vi "M266 VI Tester.vi"() -> ()   [LabVIEW 2014]
panel:
  out "Dispersion":dbl format="%.4f"
  in  "Demo mode":bool=TRUE
  out "Error":string
  out "Cur. state":i32(ring) items=["Unknown", "Open", "Close"]
  in  "Set shutter state":bool
  in  "Select shutter state":u32(ring) items=["Open", "Close"]
  out "Cur. filter":i32(ring) items=["Filter1", "Filter2", "Filter3", "Filter4", "Filter5", "Filter6", "Filter7", "Filter8"]
  in  "Set filter":bool
  in  "Select filter":i32(ring) items=["Filter1", "Filter2", "Filter3", "Filter4", "Filter5", "Filter6", "Filter7", "Filter8"]
  out "Cur. mirror":u32(ring) items=["Axial port", "Lateral port"]
  in  "Set mirror":bool
  in  "Select mirror":i32(ring) items=["Axial port", "Lateral port"]
  in  "Reset":bool
  in  "Set slit width":bool
  out "Slit width":dbl format="%.2f"
  in  "Select slit":u32(ring) items=["Entrance Slit", "Exit Slit"]
  in  "New slit width":dbl format="%.2f"
  in  "Stop control":bool
  in  "Reset":bool caption="bReset"
  in  "Set new WL":bool caption="Boolean"
  out "Cur WL":dbl format="%.2f"
  in  "New WL":dbl format="%.2f"
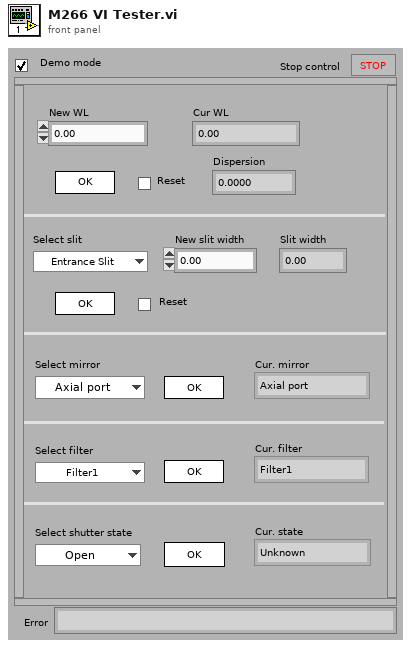
[diagram p1: front panel]
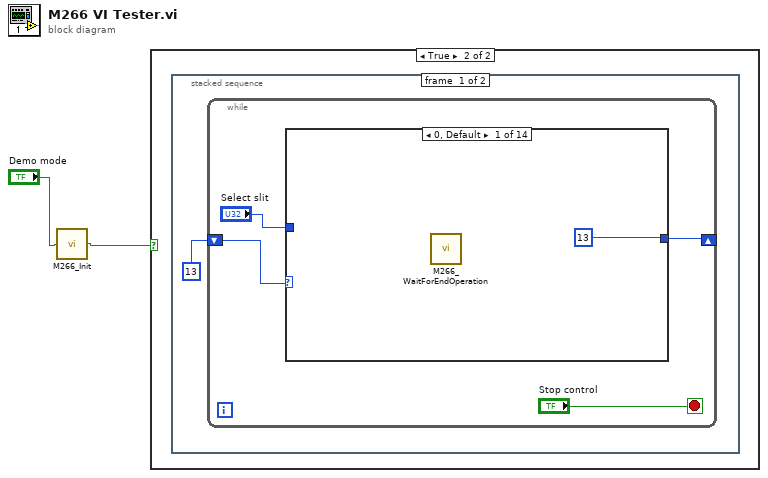
[diagram p0: block diagram]
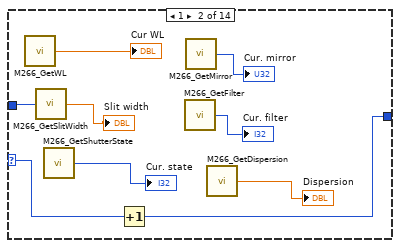
[diagram p3: hidden frame]
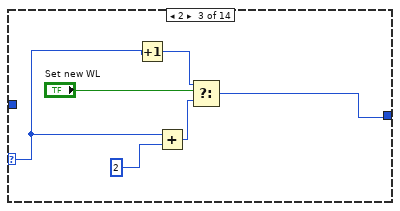
[diagram p4: hidden frame]
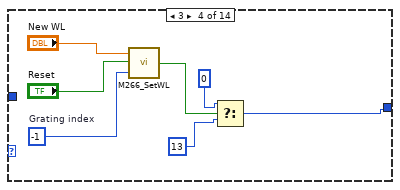
[diagram p5: hidden frame]
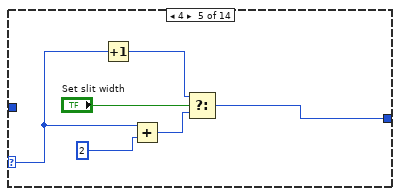
[diagram p6: hidden frame]
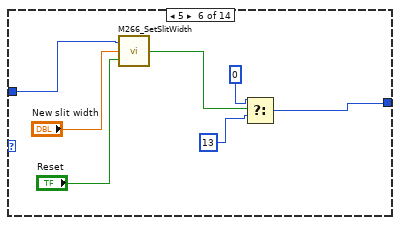
[diagram p7: hidden frame]
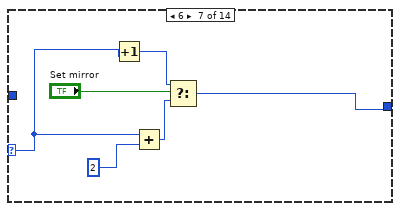
[diagram p8: hidden frame]
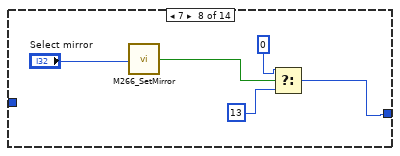
[diagram p9: hidden frame]
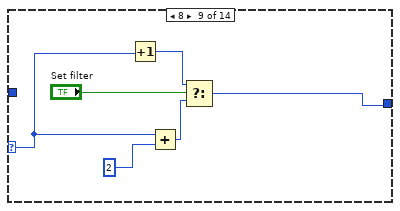
[diagram p10: hidden frame]
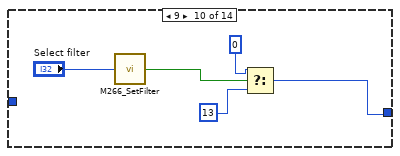
[diagram p11: hidden frame]
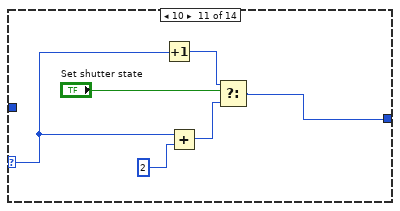
[diagram p12: hidden frame]
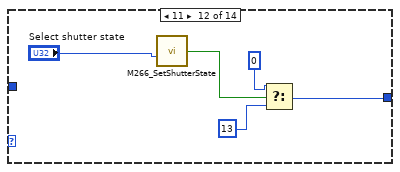
[diagram p13: hidden frame]
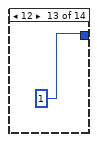
[diagram p14: hidden frame]
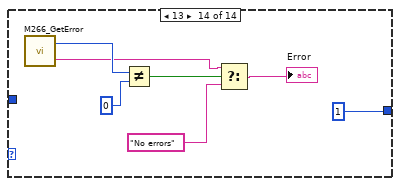
[diagram p15: hidden frame]
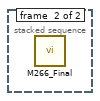
[diagram p16: hidden frame]
diagram:
  n1 = call "M266_Init.vi"("Demo mode"="Demo mode") -> ("Result"=w1:bool)
  n2 = case shown="True" w1 {
    frame False {
    }
    frame True {
      n3 = stacked-sequence {
        frame #0 {
          n4 = while {
            shift-right: [w5] -> _
            shift-left: 13 -> [w4]
            stop <- "Stop control" stop-if-true
            n5 = case shown="0, Default" w4 {
              selector: w4 -> [_ w13 w18 _ w31 _ w45 _ w56 _ w69 _ _ _]
              tunnel: "Select slit" -> [_ w15 _ _ _ w37 _ _ _ _ _ _ _ _]
              tunnel: [13 w14 w22 w25 w32 w38 w44 w51 w55 w61 w66 w73 1 1] -> w5
              frame 0, Default {
                n6 = call "M266_WaitForEndOperation.vi"() -> ()  [unwired: 1 out]
              }
              frame 1 {
                n7 = call "M266_GetWL.vi"() -> ("Current WL"=→"Cur WL":dbl)
                n8 = call "M266_GetSlitWidth.vi"("Select slit"=w15) -> ("Slit width"=→"Slit width":dbl)
                n9 = call "M266_GetShutterState.vi"() -> ("Shutter state"=→"Cur. state":i32)
                n10 = Increment(x=w13) -> (x+1=w14:i32)
                n11 = call "M266_GetFilter.vi"() -> ("Filter"=→"Cur. filter":i32)
                n12 = call "M266_GetMirror.vi"() -> ("Mirror position"=→"Cur. mirror":i32)
                n13 = call "M266_GetDispersion.vi"() -> ("Dispersion"=→"Dispersion":dbl)
              }
              frame 2 {
                n14 = Increment(x=w18) -> (x+1=w21:i32)
                n15 = Add(x=w18, y=2) -> (x+y=w19:i32)
                n16 = Select(t=w21, s="Set new WL", f=w19) -> (s? t:f=w22:i32)
              }
              frame 3 {
                w29 = -1  # Grating index
                n17 = call "M266_SetWL.vi"("Grating index"=w29, "Reset"="Reset", "WL"="New WL") -> ("Result"=w28:bool)
                n18 = Select(t=0, s=w28, f=13) -> (s? t:f=w25:i32)
              }
              frame 4 {
                n19 = Increment(x=w31) -> (x+1=w35:i32)
                n20 = Add(x=w31, y=2) -> (x+y=w34:i32)
                n21 = Select(t=w35, s="Set slit width", f=w34) -> (s? t:f=w32:i32)
              }
              frame 5 {
                n22 = call "M266_SetSlitWidth.vi"("Reset"="Reset", "Slit width"="New slit width", "Select slit"=w37) -> ("Result"=w40:bool)
                n23 = Select(t=0, s=w40, f=13) -> (s? t:f=w38:i32)
              }
              frame 6 {
                n24 = Increment(x=w45) -> (x+1=w49:i32)
                n25 = Add(x=w45, y=2) -> (x+y=w47:i32)
                n26 = Select(t=w49, s="Set mirror", f=w47) -> (s? t:f=w44:i32)
              }
              frame 7 {
                n27 = call "M266_SetMirror.vi"("Select mirror"="Select mirror") -> ("Result"=w52:bool)
                n28 = Select(t=0, s=w52, f=13) -> (s? t:f=w51:i32)
              }
              frame 8 {
                n29 = Increment(x=w56) -> (x+1=w60:i32)
                n30 = Add(x=w56, y=2) -> (x+y=w58:i32)
                n31 = Select(t=w60, s="Set filter", f=w58) -> (s? t:f=w55:i32)
              }
              frame 9 {
                n32 = call "M266_SetFilter.vi"("Select filter"="Select filter") -> ("Result"=w62:bool)
                n33 = Select(t=0, s=w62, f=13) -> (s? t:f=w61:i32)
              }
              frame 10 {
                n34 = Increment(x=w69) -> (x+1=w71:i32)
                n35 = Add(x=w69, y=2) -> (x+y=w67:i32)
                n36 = Select(t=w71, s="Set shutter state", f=w67) -> (s? t:f=w66:i32)
              }
              frame 11 {
                n37 = call "M266_SetShutterState.vi"("Select shutter state"="Select shutter state") -> ("Result"=w74:bool)
                n38 = Select(t=0, s=w74, f=13) -> (s? t:f=w73:i32)
              }
              frame 12 {
              }
              frame 13 {
                n39 = call "M266_GetError.vi"() -> ("Error text"=w79:string, "Error code"=w84:u32)
                n40 = Not Equal?(x=w84, y=0) -> (x != y?=w81:bool)
                n41 = Select(t=w79, s=w81, f="No errors") -> (s? t:f=→"Error":string)
              }
            }
          }
        }
        frame #1 {
          n42 = call "M266_Final.vi"() -> ()  [unwired: 1 in]
        }
      }
    }
  }
